vi "get power.vi"(8 "error in (no error)":errorcluster, 11 "Power Meter in":refnum<class "Power Meter.lvclass">) -> (0 "error out":errorcluster, 2 "Power":dbl=-1.0, 3 "Power Meter out":refnum<class "Power Meter.lvclass">)   [LabVIEW 2018, in "Power Meter.lvlib" / "Power Meter.lvclass"]
uses:
  Power Meter.lvclass
  C:/Program Files/National Instruments/LabVIEW 2018/vi.lib/ActorFramework/Actor/Actor.lvclass
  <vilib>/ActorFramework/Actor/Actor.lvclass/Actor.ctl
  Power Meter.lvclass/Power Meter.ctl
  Application Messages/Read Laser Power Msg/Read Laser Power Msg.lvclass/Read Laser Power Msg.ctl
  <vilib>/ActorFramework/Message Enqueuer/Message Enqueuer.lvclass/Message Enqueuer.ctl
  <vilib>/ActorFramework/Message Enqueuer/Enqueue.vi
  Application Messages/Read Laser Power Msg/Read Laser Power Msg.lvclass
  C:/Program Files/National Instruments/LabVIEW 2018/vi.lib/ActorFramework/Message/Message.lvclass
  <vilib>/ActorFramework/Message Priority Queue/Priority Enqueue.vi
  <vilib>/ActorFramework/Actor/Actor.lvclass
  Power Meter.lvlib
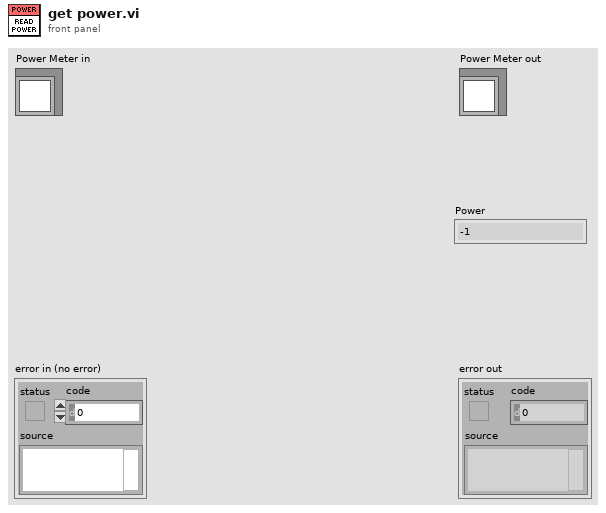
[diagram p1: front panel]
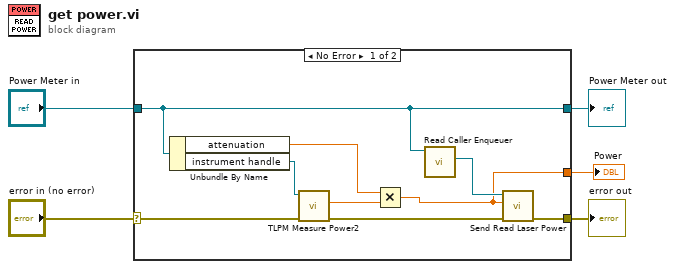
[diagram p0: block diagram]
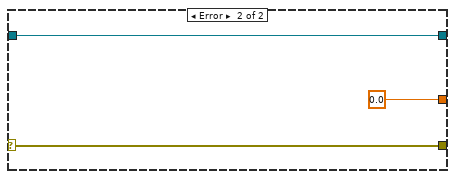
[diagram p2: hidden frame]
diagram:
  n1 = case shown="No Error" "error in (no error)" {
    selector: "error in (no error)" -> [w11 w17]
    tunnel: [w13 w17] -> w4
    tunnel: [w12 w16] -> w2
    tunnel: "Power Meter in" -> [w12 w16]
    tunnel: [w7 0.0 ("Power")] -> w1
    frame No Error {
      n2 = Unbundle By Name(w12) -> ("attenuation"=w6:dbl, "instrument handle"=w9:refnum<visa-resource-name>)
      n3 = call "TLPM Measure Power2.vi"("error in (no error)"=w11, "instrument handle"=w9) -> ("error out"=w10:errorcluster, "Power"=w8:dbl)  [unwired: 7 in, 1 out]
      n4 = Multiply(x=w6, y=w8) -> (x*y=w7:dbl)
      n5 = call <vilib>:"Read Caller Enqueuer.vi"("Actor"=w12) -> ("Caller Enqueuer"=w14:refnum<class "Message Enqueuer.lvclass">)  [unwired: 10 in]
      n6 = call "Send Read Laser Power.vi"("error in (no error)"=w10, "Power"=w7, "Message Enqueuer"=w14) -> ("error out"=w13:errorcluster)  [unwired: 7 in, 1 out]
    }
    frame Error {
    }
  }
  "error out" <- w4
  "Power Meter out" <- w2
  "Power" <- w1
